vi "Configure Scan Layer Trigger Link.vi"(7 "Scan Output Trigger Line (2: Line2)":i32(ring)=2 items=["Line1"=1, "Line2"=2, "Line3"=3, "Line4"=4, "Line5"=5, "Line6"=6], 8 "error in (no error)":errorcluster, 9 "Scan Input Trigger Line (1: Line1)":i32(ring)=1 items=["Line1"=1, "Line2"=2, "Line3"=3, "Line4"=4, "Line5"=5, "Line6"=6], 10 "Scan Source Bypass (1: Acceptor)":i32(ring)=1 items=["Source", "Acceptor"], 11 "VISA resource name":refnum<visa-resource-name>) -> (0 "error out":errorcluster, 3 "VISA resource name out":refnum<visa-resource-name>)   [LabVIEW 2019, in "Keithley 6517.lvlib"]
doc: "Sets the bypass, input trigger line and output trigger line for the Scan Layer (Arm2) of the trigger model.\n\n<B>Note:</B>\n(1)<B>Models 6517A, 6517B:</B> The trigger model consists of 3 layers, the Arm Layer, the Scan Layer (Arm2), and the Measure Layer (Trigger).\n(2)<B>Model 6514:</B> The trigger model consists of 2 layers: Arm Layer & Measure Layer (Trigger).\n\nThis VI is <B>NOT</B> compatible with model <B>6514</B>."
uses:
  Keithley 6517.lvlib
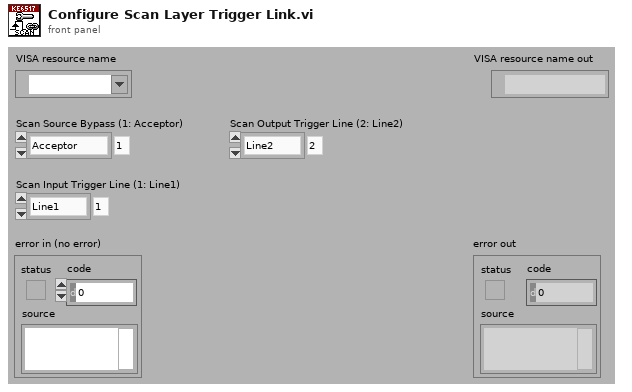
[diagram p1: front panel]
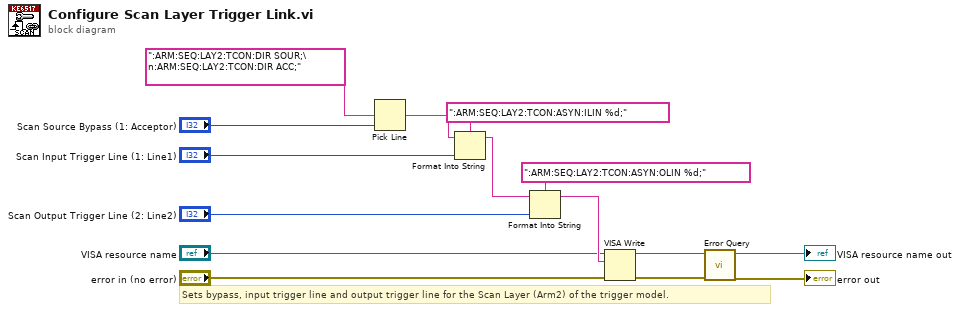
[diagram p0: block diagram]
diagram:
  # "Sets bypass, input trigger line and output trigger line for the Scan Layer (Arm2) of the trigger model."
  n1 = Pick Line(multi-line string=":ARM:SEQ:LAY2:TCON:DIR SOUR;\n:ARM:SEQ:LAY2:TCON:DIR ACC;", line index="Scan Source Bypass (1: Acceptor)") -> (output string=w1:string)  [unwired: 1 in]
  n2 = Format Into String(format string=":ARM:SEQ:LAY2:TCON:ASYN:ILIN %d;", initial string=w1, "Scan Input Trigger Line (1: Line1)") -> (resulting string=w13:string)  [unwired: 1 in, 1 out]
  n3 = Format Into String(format string=":ARM:SEQ:LAY2:TCON:ASYN:OLIN %d;", initial string=w13, "Scan Output Trigger Line (2: Line2)") -> (resulting string=w10:string)  [unwired: 1 in, 1 out]
  n4 = VISA Write(VISA resource name="VISA resource name", write buffer=w10, error in (no error)="error in (no error)") -> (VISA resource name out=w7:refnum<visa-resource-name>, error out=w6:errorcluster)  [unwired: 1 out]
  n5 = call "Error Query.vi"("error in (no error)"=w6, "VISA resource name"=w7) -> ("error out"=→"error out":errorcluster, "VISA resource name out"=→"VISA resource name out":refnum<visa-resource-name>)  [unwired: 6 in, 2 out]
